vi "DigitalDisplay.vi"(10 "外观":cluster{"小数位数":u8, "字体颜色":u32, "背景颜色":u32}={"小数位数"=2, "字体颜色"=6618880, "背景颜色"=0}, 11 "通道选择":string[](array[string])) -> ()   [LabVIEW 2018, in "DataDisplay.lvlib"]
doc: "(<B>Filename</B>: Actor Framework.lvlib:Actor.lvclass:Actor Core.vi)\n\nReceives messages to the actor, reacts to them, and initiates any error handling that may shut the actor down.\n\nDescendant classes may override this VI to append parallel tasks for the actor to complete while it handles messages. Overrides use the Call Parent Method node."
uses:
  DataDisplay.lvlib
  DigitalDisplay/DigitalDisplay.lvclass
  DigitalDisplay/DigitalDisplayRef.ctl
  TypeDefine/DD_DataStream.ctl
  SubVI/DD_Parameter.vi
panel:
  in  "显示数组":cluster{"通道选择":u16, "数值":string}[](array[cluster]) {"通道选择" items=["位移1 [mm]", "力1 [mm]", "次数1 [次]", "位移2 [mm]", "力2 [mm]", "次数2 [次]"]}
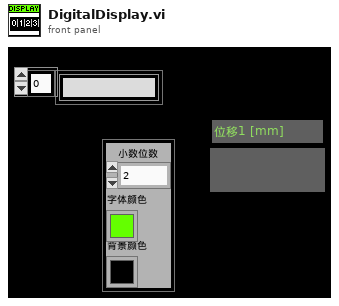
[diagram p1: front panel]
types:
  T1 = typedef "DataDisplay.lvlib/DigitalDisplay.lvclass/DigitalDisplayRef.ctl" = cluster{"r显示数组":refnum<vi>, "r显示单元":refnum<vi>, "r通道选择":refnum<vi>, "r数值":refnum<vi>, "rVI":refnum<vi>, "rPane":refnum<vi>, "DD_数据通知器":refnum<notifier>}
  T2 = typedef "LVPoint32TypeDef.ctl" = cluster{"Horizontal":i32, "Vertical":i32}
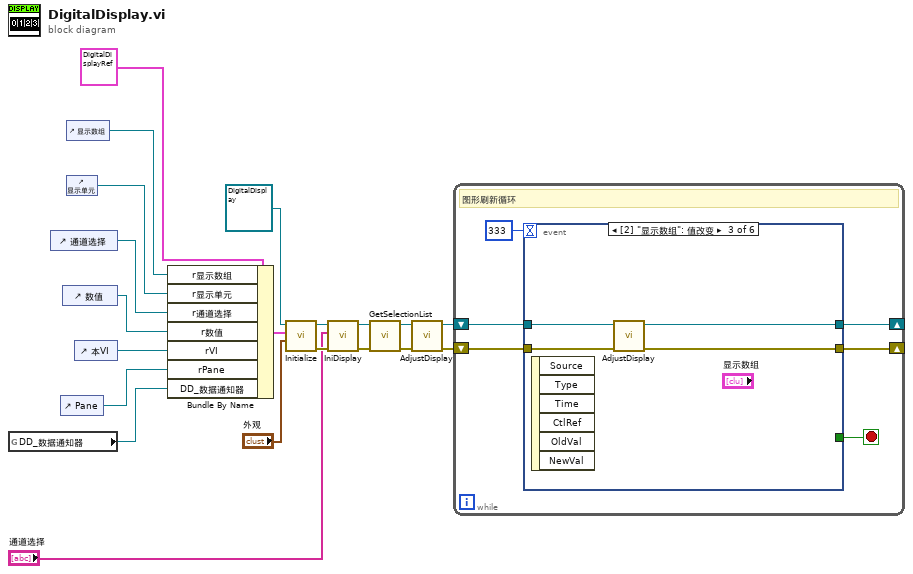
[diagram p0: block diagram]
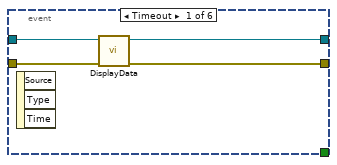
[diagram p2: hidden frame]
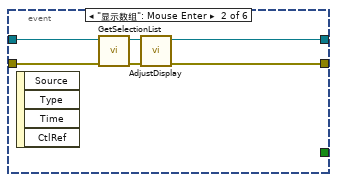
[diagram p3: hidden frame]
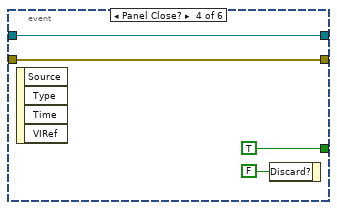
[diagram p4: hidden frame]
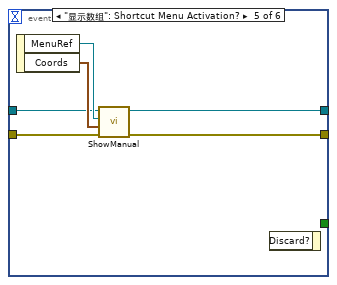
[diagram p5: hidden frame]
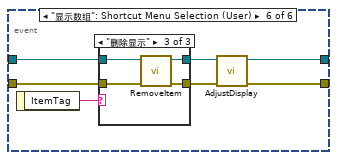
[diagram p6: hidden frame]
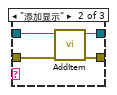
[diagram p8: hidden frame]
diagram:
  n1 = global read "DD_Parameter.vi" "DD_数据通知器"() -> (w12:refnum<notifier>)
  n2 = control-ref of="通道选择"() -> (w17:refnum<vi>)
  n3 = control-ref of="Pane"() -> (w13:refnum<vi>)
  n4 = control-ref of="数值"() -> (w18:refnum<vi>)
  n5 = control-ref of="显示数组"() -> (w15:refnum<vi>)
  n6 = control-ref of="显示单元"() -> (w16:refnum<vi>)
  n7 = control-ref of="本VI"() -> (w14:refnum<vi>)
  n8 = Bundle By Name(cluster=T1 {"r显示数组"=refnum, "r显示单元"=refnum, "r通道选择"=refnum, "r数值"=refnum, "rVI"=refnum, "rPane"=refnum, "DD_数据通知器"=refnum} ("引用"), "r显示数组"=w15, "r显示单元"=w16, "r通道选择"=w17, "r数值"=w18, "rVI"=w14, "rPane"=w13, "DD_数据通知器"=w12) -> (w11:T1)
  n9 = call "Initialize.vi"("外观"="外观", "引用"=w11, "DigitalDisplay 输入"=refnum<class "DigitalDisplay.lvclass"> refnum ("DigitalDisplay.lvclass")) -> ("error out"=w6:errorcluster, "DigitalDisplay 输出"=w9:refnum<class "DigitalDisplay.lvclass">)  [unwired: 7 in]
  n10 = call "IniDisplay.vi"("error in (no error)"=w6, "通道选择"="通道选择", "DigitalDisplay 输入"=w9) -> ("error out"=w5:errorcluster, "DigitalDisplay 输出"=w8:refnum<class "DigitalDisplay.lvclass">)  [unwired: 7 in]
  n11 = call "GetSelectionList.vi"("error in (no error)"=w5, "DigitalDisplay 输入"=w8) -> ("error out"=w4:errorcluster, "DigitalDisplay 输出"=w7:refnum<class "DigitalDisplay.lvclass">)  [unwired: 8 in]
  n12 = call "AdjustDisplay.vi"("error in (no error)"=w4, "DigitalDisplay 输入"=w7) -> ("error out"=w2:errorcluster, "DigitalDisplay 输出"=w3:refnum<class "DigitalDisplay.lvclass">)  [unwired: 8 in]
  n13 = while {
    shift-right: [w22] -> _
    shift-left: w3 -> [w24]
    shift-right: [w21] -> _
    shift-left: w2 -> [w23]
    stop <- w25 stop-if-true
    # "图形刷新循环"
    n14 = event shown="[2] \"显示数组\": 值改变" {
      selector: _ -> [_ _ _ _ _ _]
      dyn-events: _ -> [_ _ _ _ _ _]
      timeout: 333 -> [_ _ _ _ _ _]
      tunnel: [_ _ _ TRUE _ _] -> w25
      tunnel: w24 -> [w30 w36 w40 w42 w47 w56]
      tunnel: w23 -> [w28 w35 w39 w41 w48 w55]
      tunnel: [w29 w33 w38 w42 w46 w52] -> w22
      tunnel: [w27 w31 w37 w41 w45 w51] -> w21
      event Timeout {
        n15 = event-data() -> ()  [unwired: 1 in, 3 out]
        n16 = call "DisplayData.vi"("error in (no error)"=w28, "DigitalDisplay 输入"=w30) -> ("error out"=w27:errorcluster, "DigitalDisplay 输出"=w29:refnum<class "DigitalDisplay.lvclass">)  [unwired: 8 in]
      }
      event "显示数组": Mouse Enter {
        n17 = event-data() -> ()  [unwired: 1 in, 4 out]
        n18 = call "GetSelectionList.vi"("error in (no error)"=w35, "DigitalDisplay 输入"=w36) -> ("error out"=w32:errorcluster, "DigitalDisplay 输出"=w34:refnum<class "DigitalDisplay.lvclass">)  [unwired: 8 in]
        n19 = call "AdjustDisplay.vi"("error in (no error)"=w32, "DigitalDisplay 输入"=w34) -> ("error out"=w31:errorcluster, "DigitalDisplay 输出"=w33:refnum<class "DigitalDisplay.lvclass">)  [unwired: 8 in]
      }
      event "显示数组": Value Change {
        n20 = event-data() -> ()  [unwired: 1 in, 6 out]
        n21 = call "AdjustDisplay.vi"("error in (no error)"=w39, "DigitalDisplay 输入"=w40) -> ("error out"=w37:errorcluster, "DigitalDisplay 输出"=w38:refnum<class "DigitalDisplay.lvclass">)  [unwired: 8 in]
      }
      event Panel Close? {
        n22 = event-data() -> ()  [unwired: 1 in, 4 out]
        n23 = event-data("Discard?"=FALSE ("放弃？")) -> ()  [unwired: 1 in, 1 out]
      }
      event "显示数组": Shortcut Menu Activation? {
        n24 = event-data() -> ("MenuRef"=w49:refnum<k9>, "Coords"=w50:T2)  [unwired: 1 in]
        n25 = call "ShowManual.vi"("error in (no error)"=w48, "坐标"=w50, "菜单引用"=w49, "DigitalDisplay 输入"=w47) -> ("error out"=w45:errorcluster, "DigitalDisplay 输出"=w46:refnum<class "DigitalDisplay.lvclass">)  [unwired: 6 in]
        n26 = event-data() -> ()  [unwired: 2 in, 1 out]
      }
      event "显示数组": Shortcut Menu Selection (User) {
        n27 = event-data() -> ("ItemTag"=w57:string)  [unwired: 1 in]
        n28 = case shown="\"删除显示\"" w57 {
          tunnel: w56 -> [w59 w63 w67]
          tunnel: w55 -> [w58 w62 w66]
          tunnel: [w59 w61 w64] -> w54
          tunnel: [w58 w60 w65] -> w53
          frame "假", Default {
          }
          frame "添加显示" {
            n29 = call "AddItem.vi"("error in (no error)"=w62, "DigitalDisplay 输入"=w63) -> ("error out"=w60:errorcluster, "DigitalDisplay 输出"=w61:refnum<class "DigitalDisplay.lvclass">)  [unwired: 8 in]
          }
          frame "删除显示" {
            n30 = call "RemoveItem.vi"("error in (no error)"=w66, "DigitalDisplay 输入"=w67) -> ("error out"=w65:errorcluster, "DigitalDisplay 输出"=w64:refnum<class "DigitalDisplay.lvclass">)  [unwired: 8 in]
          }
        }
        n31 = call "AdjustDisplay.vi"("error in (no error)"=w53, "DigitalDisplay 输入"=w54) -> ("error out"=w51:errorcluster, "DigitalDisplay 输出"=w52:refnum<class "DigitalDisplay.lvclass">)  [unwired: 8 in]
      }
    }
  }
